vi "Set Target Names.vi"(8 "error in":errorcluster, 11 "DIG_IO in":refnum<class "DIG_IO.lvclass">) -> (0 "error out":errorcluster, 3 "DIG_IO out":refnum<class "DIG_IO.lvclass">)   [LabVIEW 2019, in "DIG_IO.lvlib" / "DIG_IO.lvclass"]
uses:
  Library/DIG_IO.lvclass
  Library/DIG_IO.lvclass/DIG_IO.ctl
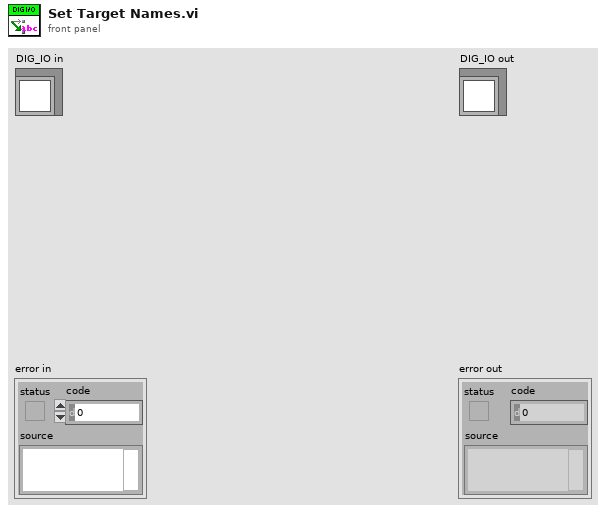
[diagram p1: front panel]
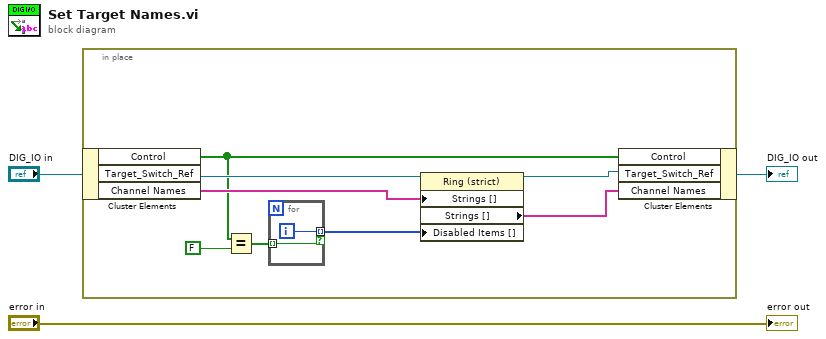
[diagram p0: block diagram]
diagram:
  n1 = in-place {
    n2 = in-place-cluster #1("DIG_IO in") -> ("Control"=w5:bool[], "Target_Switch_Ref"=w11:refnum<vi>, "Channel Names"=w10:string[])
    n3 = Equal?(x=w5, y=FALSE) -> (x = y?=w6:bool[])
    n4 = for {
      tunnel: w6 -> [w12] mode=indexing
      tunnel: [w13] -> w4 mode=indexing if=w12
      i -> [w13]
    }
    n5 = property class="Ring (strict)"(reference=w11, "Strings []"=w10, "Disabled Items []"=w4) -> (reference out=w8:refnum<vi>, "Strings []"=w9:string[])  [unwired: 1 in, 1 out]
    n6 = in-place-cluster #1("Control"=w5, "Target_Switch_Ref"=w8, "Channel Names"=w9) -> (→"DIG_IO out":refnum<class "DIG_IO.lvclass">)
  }
  "error out" <- "error in"
